vi "TextShowAdd2End.vi"(10 "TxtAdd":string, 11 "TxtBox":refnum<vi>) -> ()   [LabVIEW 2016]
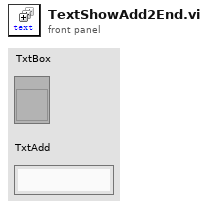
[diagram p1: front panel]
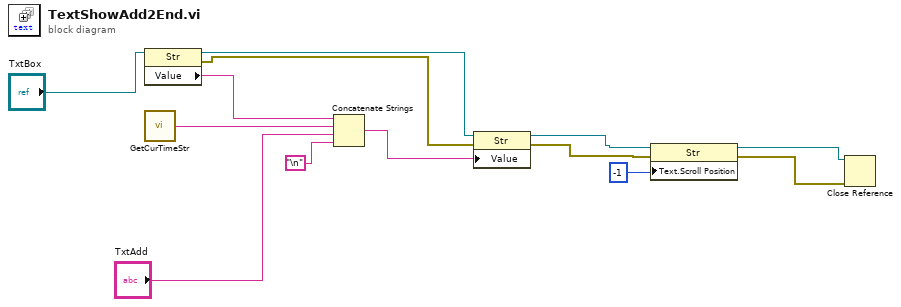
[diagram p0: block diagram]
diagram:
  n1 = property class="Str"(reference="TxtBox") -> (reference out=w7:refnum<vi>, error out=w2:errorcluster, "Value"=w10:string)  [unwired: 1 in]
  n2 = call "GetCurTimeStr.vi"() -> ("Time"=w11:string)  [unwired: 3 in]
  n3 = Concatenate Strings(w10, w11, "TxtAdd", "\n") -> (w13:string)
  n4 = property class="Str"(reference=w7, error in=w2, "Value"=w13) -> (reference out=w4:refnum<vi>, error out=w3:errorcluster)
  n5 = property class="Str"(reference=w4, error in=w3, "Text.Scroll Position"=-1 ("文本.滚动条位置")) -> (reference out=w5:refnum<vi>, error out=w1:errorcluster)
  n6 = Close Reference(reference=w5, error in (no error)=w1) -> ()  [unwired: 1 out]
